vi "Display.vi"(8 "error in":errorcluster, 11 "Input (DBL) in":refnum<class "GIF - Input (DBL).lvclass">) -> (0 "error out":errorcluster, 3 "Input (DBL) out":refnum<class "GIF - Input (DBL).lvclass">)   [LabVIEW 2021, in "GIF - Input (DBL).lvclass"]
doc: "This vi will display the input pop up waiting for a type Double input from the user\n\nThe graphic will be an input from the developer.\n\n<b>Code Developed By:</b>\nDaniel Coons\nTechnology Service Corporation\n1983 S Liberty Drive\nBloomington, IN 47403\nPhone: 812 558-7100\ndaniel.coons@tsc.com\nwww.tsc.com/atcs"
uses:
  GIF - Input (DBL).lvclass
  C:/Program Files/National Instruments/LabVIEW 2024/vi.lib/addons/_TSC/TSC Pop-Up/Popup/Popup.lvclass
  C:/Development/tsc-pop-up-gif/GIF Parent.lvclass
  GIF - Input (DBL).lvclass/GIF - Input (DBL).ctl
  <vilib>/addons/_TSC/TSC Pop-Up/Popup/Popup.lvclass/Popup.ctl
  GIF Parent.lvclass/GIF Parent.ctl
  <vilib>/addons/_TSC/TSC Pop-Up/Popup/Data Member Access/Read Theme.vi
  Read Delays.vi
  Read Gif Images.vi
  <vilib>/addons/_TSC/TSC Pop-Up/Theme/Theme.lvclass
  <vilib>/addons/_TSC/TSC Pop-Up/Popup/Popup.lvclass
  user32.dll
panel:
  in  "closer":bool
  out "header":bool
  in  "OK":bool
  out "Input value out":dbl=1.0 min=1.0
  out "2D Picture":picture
  out "Message":string
  in  "Input":dbl
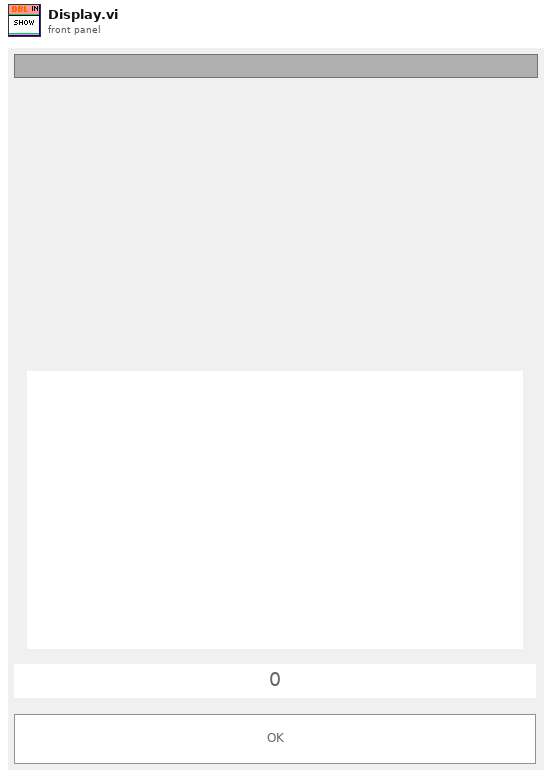
[diagram p1: front panel]
types:
  T1 = typedef "LVPoint32TypeDef.ctl" = cluster{"Horizontal":i32, "Vertical":i32}
  T2 = typedef "LVPositionTypeDef.ctl" = cluster{"Left":i32, "Top":i32}
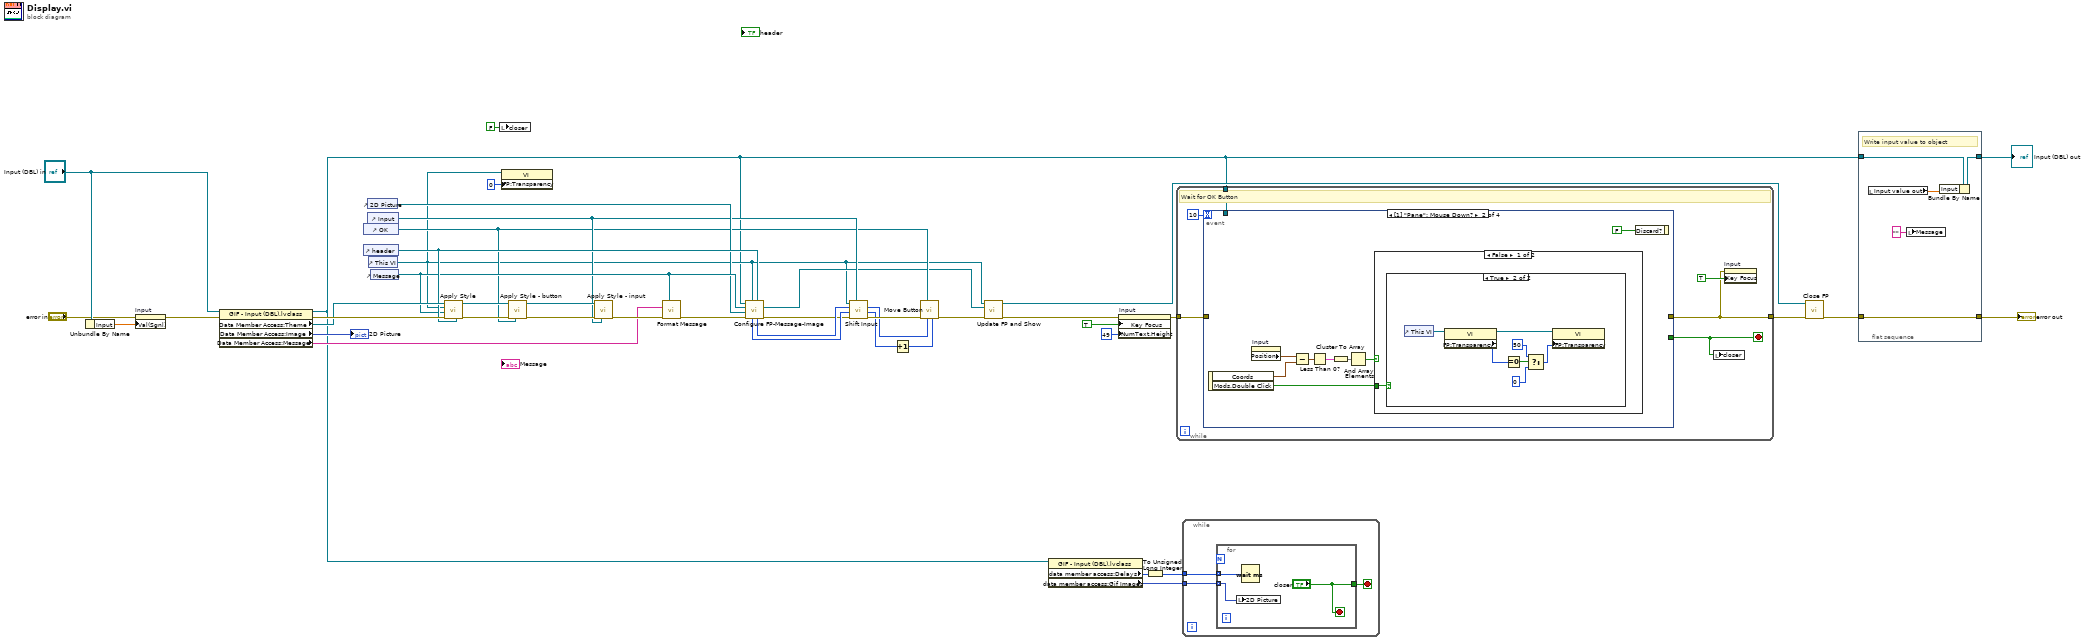
[diagram p0: block diagram]
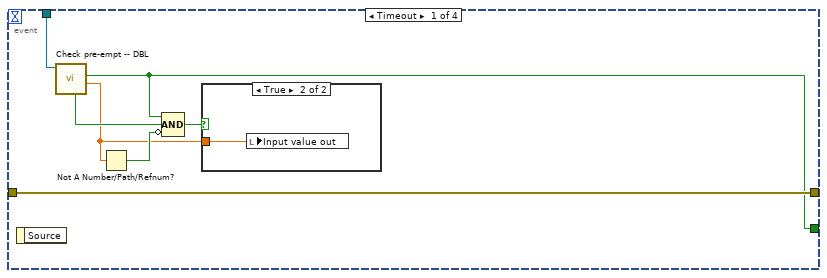
[diagram p2: hidden frame]
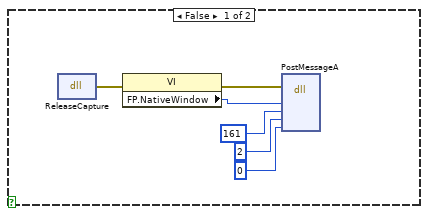
[diagram p4: hidden frame]
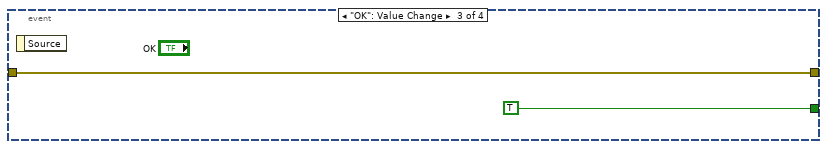
[diagram p6: hidden frame]
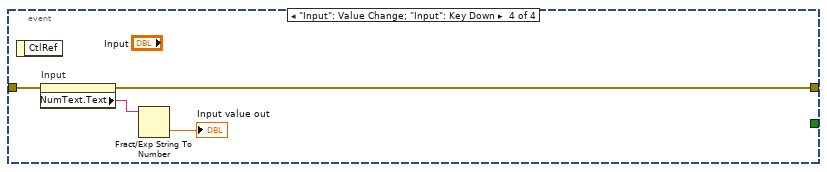
[diagram p7: hidden frame]
diagram:
  n1 = Unbundle By Name("Input (DBL) in") -> ("Input"=w39:dbl)
  n2 = property on="Input" class="DigNum (strict)"(error in="error in", "Val(Sgnl)"=w39) -> (error out=w40:errorcluster)  [unwired: 1 in, 1 out]
  n3 = property class="GIF - Input (DBL).lvclass"(reference="Input (DBL) in", error in=w40) -> (reference out=w2:refnum<class "GIF - Input (DBL).lvclass">, error out=w19:errorcluster, "Data Member Access:Theme"=w17:refnum<class "Theme.lvclass">, "Data Member Access:Image"=→"2D Picture":picture, "Data Member Access:Message"=w18:string)
  n4 = control-ref of="OK"() -> (w12:refnum<vi>)
  n5 = control-ref of="header"() -> (w16:refnum<vi>)
  n6 = control-ref of="2D Picture"() -> (w14:refnum<vi>)
  n7 = control-ref of="Input"() -> (w13:refnum<vi>)
  n8 = control-ref of="This VI"() -> (w6:refnum<vi>)
  n9 = control-ref of="Message"() -> (w15:refnum<vi>)
  n10 = call <vilib>:"Apply Style.vi"("header ref"=w16, "error in (no error)"=w19, "message ref"=w15, "pop up ref"=w6, "Theme in"=w17) -> ("error out"=w31:errorcluster, "Theme out"=w28:refnum<class "Theme.lvclass">)  [unwired: 5 in]
  n11 = local write "closer"(FALSE ("closer")) -> ()
  n12 = property on="Property Node" class="VI"(reference=w6, "FP:Transparency"=u8 0 ("Front Panel Window:Transparency")) -> ()  [unwired: 1 in, 2 out]
  n13 = call <vilib>:"Apply Style - button.vi"("button ref"=w12, "error in (no error)"=w31, "Theme in"=w28) -> ("error out"=w30:errorcluster, "Theme out"=w27:refnum<class "Theme.lvclass">)  [unwired: 7 in]
  n14 = call <vilib>:"Apply Style - input.vi"("input ref"=w13, "error in (no error)"=w30, "Theme in"=w27) -> ("error out"=w29:errorcluster)  [unwired: 7 in, 1 out]
  n15 = call <vilib>:"Format Message.vi"("formatted string"=w15, "error in"=w29, "String Input"=w18) -> ("error out"=w32:errorcluster)  [unwired: 7 in, 1 out]
  n16 = call <vilib>:"Configure FP-Message-Image.vi"("header ref"=w16, "Pop Up ref"=w6, "error in (no error)"=w32, "Image ref"=w14, "Message ref"=w15, "Popup in"=w2) -> ("error out"=w21:errorcluster, "Panel Ref"=w11:refnum<vi>, "Panel Width"=w23:i32, "Panel Height"=w22:i32)  [unwired: 1 in, 1 out]
  n17 = call <vilib>:"Shift Input.vi"("Control"=w13, "Error In"=w21, "Panel Height"=w22, "Panel Width"=w23, "Pop Up ref"=w6) -> ("Error Out"=w26:errorcluster, "Panel Height out"=w10:i32, "Panel Width out"=w25:i32)  [unwired: 4 in]
  n18 = Increment(x=w10) -> (x+1=w24:i32)
  n19 = call <vilib>:"Move Button.vi"("Panel Height"=w24, "Panel Width"=w25, "Button"=w12, "Error In"=w26) -> ("Error Out"=w20:errorcluster)  [unwired: 6 in, 1 out]
  n20 = call <vilib>:"Update FP and Show.vi"("error in (no error)"=w20, "Panel Ref"=w11, "VI in"=w6) -> ("error out"=w36:errorcluster, "VI out"=w7:refnum<vi>)  [unwired: 7 in]
  n21 = property class="GIF - Input (DBL).lvclass"(reference=w2) -> ("data member access:Delays"=w5:i32[], "data member access:Gif Images"=w4:picture[])  [unwired: 1 in, 2 out]
  n22 = property on="Input" class="DigNum (strict)"(error in=w36, "Key Focus"=TRUE, "NumText.Height"=u32 49 ("Numeric Text.Size:Height")) -> (error out=w35:errorcluster)  [unwired: 1 in, 1 out]
  n23 = To Unsigned Long Integer(number=w5) -> (unsigned 32bit integer=w3:u32[])
  n24 = while {
    tunnel: w35 -> [w50]
    tunnel: [w46] -> w38
    tunnel: w2 -> [w48]
    stop <- w45 stop-if-true
    # "Wait for OK Button"
    n25 = event shown="[1] \"Pane\": Mouse Down?" {
      selector: _ -> [_ _ _ _]
      dyn-events: _ -> [_ _ _ _]
      timeout: 10 -> [_ _ _ _]
      tunnel: w50 -> [w57 _ w82 w86]
      tunnel: [w57 _ w82 w84] -> w46
      tunnel: [w52 _ TRUE _] -> w45
      tunnel: w48 -> [w51 _ _ _]
      event Timeout {
        n26 = event-data() -> ()  [unwired: 1 in, 1 out]
        n27 = call <vilib>:"Check pre-empt -- DBL.vi"("_Popup in"=w51) -> ("Value?"=w53:dbl, "Pre-empted?"=w52:bool, "Type Match?"=w55:bool)  [unwired: 7 in, 1 out]
        n28 = Not A Number/Path/Refnum?(number/path/refnum=w53) -> (NaN/Path/Refnum?=w56:bool)
        n29 = Compound Arithmetic op=AND(w52, w55, invert w56) -> (w54:bool)
        n30 = case shown="True" w54 {
          tunnel: w53 -> [_ w58]
          frame False {
          }
          frame True {
            n31 = local write "Input value out"(w58) -> ()
          }
        }
      }
      event Mouse Down? {
        n32 = event-data() -> ("Coords"=w60:T1, "Mods.Double Click"=w59:bool)  [unwired: 1 in]
        n33 = property on="Input" class="DigNum (strict)"() -> ("Position"=w65:T2)  [unwired: 2 in, 2 out]
        n34 = Subtract(x=w65, y=w60) -> (x-y=w64:T2)
        n35 = Less Than 0?(x=w64) -> (x < 0?=w63:cluster{"Left":bool, "Top":bool})
        n36 = Cluster To Array(cluster=w63) -> (array=w62:bool[])
        n37 = And Array Elements(Boolean array=w62) -> (logical AND=w61:bool)
        n38 = case shown="False" w61 {
          tunnel: w59 -> [w67 _]
          frame False {
            n39 = case shown="True" w67 {
              frame False {
                n40 = dll-call lib="user32.dll" fn="ReleaseCapture"() -> (error out=w71:errorcluster)  [unwired: 4 in, 1 out]
                n41 = property class="VI"(error in=w71) -> (error out=w72:errorcluster, "FP.NativeWindow"=w73:u64)  [unwired: 1 in, 1 out]
                n42 = dll-call lib="user32.dll" fn="PostMessageA"(error in=w72, "hWnd"=w73, "Msg"=161, "wParam"=2, "lParam"=0) -> ()  [unwired: 7 in, 2 out]
              }
              frame True {
                n43 = control-ref of="This VI"() -> (w80:refnum<vi>)
                n44 = property class="VI"(reference=w80) -> (reference out=w78:refnum<vi>, "FP:Transparency"=w79:u8)  [unwired: 1 in, 1 out]
                n45 = Equal To 0?(x=w79) -> (x = 0?=w77:bool)
                n46 = Select(t=u8 50, s=w77, f=u8 0) -> (s? t:f=w76:u8)
                n47 = property class="VI"(reference=w78, "FP:Transparency"=w76) -> ()  [unwired: 1 in, 2 out]
              }
            }
          }
          frame True {
          }
        }
        n48 = event-data("Discard?"=FALSE) -> ()  [unwired: 1 in, 1 out]
      }
      event "OK": Value Change {
        n49 = event-data() -> ()  [unwired: 1 in, 1 out]
      }
      event "Input": Value Change; "Input": Key Down {
        n50 = event-data() -> ()  [unwired: 1 in, 1 out]
        n51 = property on="Input" class="DigNum (strict)"(error in=w86) -> (error out=w84:errorcluster, "NumText.Text"=w85:string)  [unwired: 1 in, 1 out]
        n52 = Fract/Exp String To Number(string=w85) -> (number=→"Input value out":dbl)  [unwired: 3 in, 1 out]
      }
    }
    n53 = local write "closer"(w45) -> ()
    n54 = property on="Input" class="DigNum (strict)"(error in=w46, "Key Focus"=TRUE) -> ()  [unwired: 1 in, 2 out]
  }
  n55 = while {
    tunnel: w3 -> [w88]
    tunnel: w4 -> [w87]
    stop <- w89 stop-if-true
    n56 = for {
      tunnel: ["closer"] -> w89
      tunnel: w88 -> [w91] mode=indexing
      tunnel: w87 -> [w90] mode=indexing
      stop <- "closer" stop-if-true
      n57 = local write "2D Picture"(w90) -> ()
      n58 = Wait (ms)(milliseconds to wait=w91) -> ()  [unwired: 1 out]
    }
  }
  n59 = call <vilib>:"Close FP.vi"("error in (no error)"=w38, "VI in"=w7) -> ("error out"=w37:errorcluster)  [unwired: 9 in]
  n60 = flat-sequence {
    tunnel: w37 -> [w97]
    tunnel: [w97] -> w41
    tunnel: w2 -> [w96]
    tunnel: [w95] -> w42
    frame #0 {
      # "Write input value to object"
      n61 = local read "Input value out"() -> (w94:dbl)
      n62 = local write "Message"("" ("Message")) -> ()
      n63 = Bundle By Name(cluster=w96, "Input"=w94) -> (w95:refnum<class "GIF - Input (DBL).lvclass">)
    }
  }
  "error out" <- w41
  "Input (DBL) out" <- w42
